vi "DocRoot Folder.vi"(3 "Relative Path (\"\" - Folder)":string) -> (1 "DocumentRoot Folder":path)   [LabVIEW 2011]
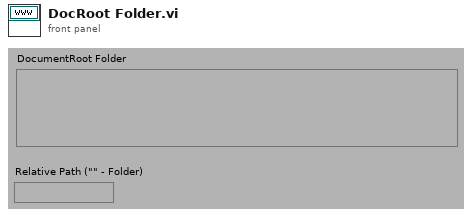
[diagram p1: front panel]
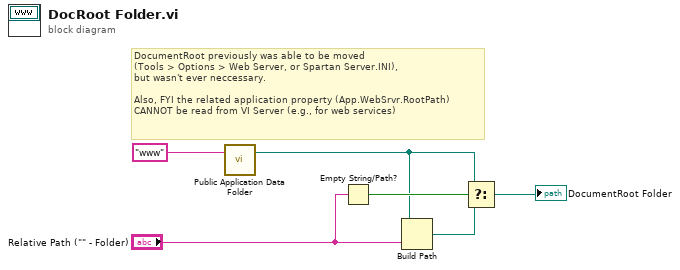
[diagram p0: block diagram]
diagram:
  # "DocumentRoot previously was able to be moved\n(Tools > Options > Web Server, or Spartan Server.INI), \nbut wasn't ever neccessary.\n\nAlso, FYI the related application property (App.WebSrvr.RootPath) \nCANNOT be read from VI Server (e.g., for web services)"
  n1 = call "Public Application Data Folder.vi"("Relative Path (\"\" - Folder)"="www") -> ("Client Storage Path"=w1:path)  [unwired: 2 in]
  n2 = Empty String/Path?(string/path="Relative Path (\"\" - Folder)") -> (empty?=w6:bool)
  n3 = Build Path(base path=w1, name or relative path="Relative Path (\"\" - Folder)") -> (appended path=w5:path)
  n4 = Select(t=w1, s=w6, f=w5) -> (s? t:f=→"DocumentRoot Folder":path)
